vi "test Path String and Path Array Functions.vi"(8 "error in (no error)":errorcluster, 11 "TestCase in":refnum<class "Variant Data Manipulation Tests.lvclass">) -> (0 "error out":errorcluster, 3 "TestCase out":refnum<class "Variant Data Manipulation Tests.lvclass">)   [LabVIEW 2017, in "Variant Data Manipulation Tests.lvclass"]
uses:
  Variant Data Manipulation Tests.lvclass
  <vilib>/addons/_JKI Toolkits/VI Tester/TestCase.llb/TestCase.lvclass
  Source/Variant Data Manipulation.lvlib
  C:/Program Files (x86)/National Instruments/LabVIEW 2017/vi.lib/addons/_JKI Toolkits/VI Tester/TestCase.llb/TestCase.lvclass
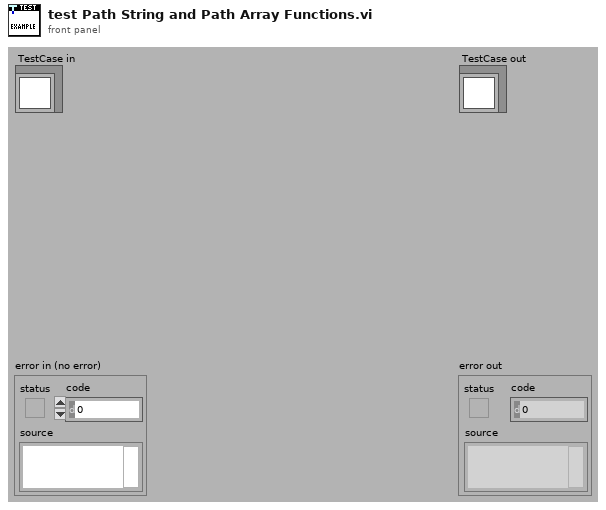
[diagram p1: front panel]
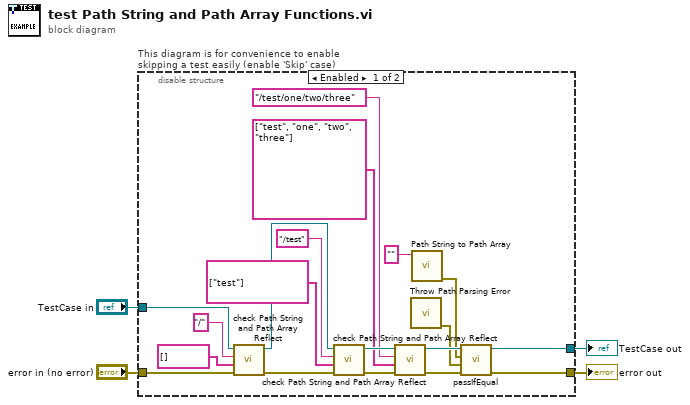
[diagram p0: block diagram]
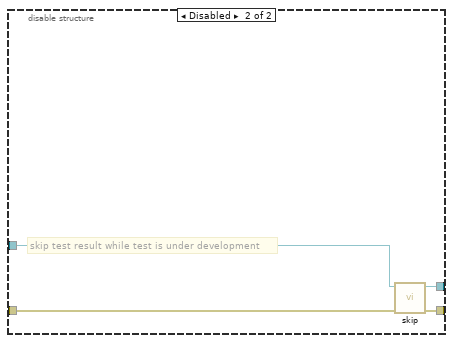
[diagram p2: hidden frame]
diagram:
  n1 = disable-structure "This diagram is for convenience to enable skipping a test easily (enable 'Skip' case)" shown="Enabled" {
    disable-tunnel: "TestCase in" -> [w23 w27]
    disable-tunnel: [w9 w25] -> w1
    disable-tunnel: [w6 w26] -> w3
    disable-tunnel: "error in (no error)" -> [w22 w24]
    frame Enabled {
      n2 = call "check Path String and Path Array Reflect.vi"("error in (no error)"=w22, "Array"=string[] [], "String"="/", "Variant Data Manipulation Tests in"=w23) -> ("error out"=w20:errorcluster, "Variant Data Manipulation Tests out"=w17:refnum<class "Variant Data Manipulation Tests.lvclass">)  [unwired: 6 in]
      n3 = call "check Path String and Path Array Reflect.vi"("error in (no error)"=w20, "Array"=string[] ["test"], "String"="/test", "Variant Data Manipulation Tests in"=w17) -> ("error out"=w18:errorcluster, "Variant Data Manipulation Tests out"=w14:refnum<class "Variant Data Manipulation Tests.lvclass">)  [unwired: 6 in]
      n4 = call "check Path String and Path Array Reflect.vi"("error in (no error)"=w18, "Array"=string[] ["test", "one", "two", "three"], "String"="/test/one/two/three", "Variant Data Manipulation Tests in"=w14) -> ("error out"=w5:errorcluster, "Variant Data Manipulation Tests out"=w13:refnum<class "Variant Data Manipulation Tests.lvclass">)  [unwired: 6 in]
      n5 = call "Throw Path Parsing Error.vi"() -> ("error out"=w7:errorcluster)  [unwired: 11 in]
      n6 = call "Path String to Path Array.vi"("Path String"="") -> ("error out"=w8:errorcluster)  [unwired: 9 in, 1 out]
      n7 = call-dynamic "passIfEqual.vi"("error in (no error)"=w5, "y"=w7, "x"=w8, "TestCase in"=w13) -> ("error out"=w6:errorcluster, "TestCase out"=w9:refnum<class "Variant Data Manipulation Tests.lvclass">)  [unwired: 6 in]
    }
    frame Disabled {
      # "skip test result while test is under development"
      n8 = call <vilib>:"skip.vi"("error in (no error)"=w24, "TestCase in"=w27) -> ("error out"=w26:errorcluster, "TestCase out"=w25:refnum<class "Variant Data Manipulation Tests.lvclass">)  [unwired: 8 in]
    }
  }
  "error out" <- w3
  "TestCase out" <- w1
